vi "publishSummaryStateEvent.vi"(8 "error in (no error)":errorcluster, 11 "Model in":refnum<class "Model.lvclass">) -> (0 "error out":errorcluster, 3 "Model out":refnum<class "Model.lvclass">)   [LabVIEW 2016, in "Model.lvclass"]
uses:
  Model.lvclass
  Communicator/Topics/EventSummaryState.ctl
  Types/Timestamp.ctl
  Types/SummaryStates.ctl
  Model.lvclass/Model.ctl
  Communicator/Communicator/Communicator.lvclass
  Types/M1M3SupportTypes.lvlib
  Communicator/M1M3Communicator.lvlib
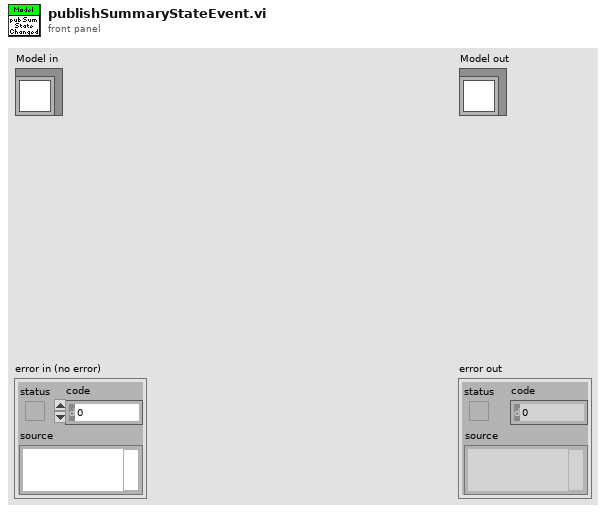
[diagram p1: front panel]
types:
  T1 = typedef "M1M3Communicator.lvlib/EventSummaryState.ctl" = cluster{"Timestamp":T2, "SummaryStates":T3}
  T2 = typedef "M1M3SupportTypes.lvlib/Timestamp.ctl" = dbl
  T3 = typedef "M1M3SupportTypes.lvlib/SummaryStates.ctl" = enum16{"OfflineState", "StandbyState", "DisabledState", "EnabledState", "FaultState"}
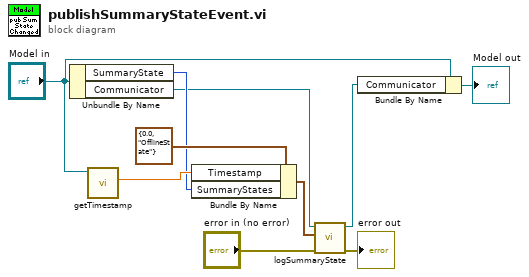
[diagram p0: block diagram]
diagram:
  n1 = Unbundle By Name("Model in") -> ("SummaryState"=w8:T3, "Communicator"=w7:refnum<class "Communicator.lvclass">)
  n2 = call "getTimestamp.vi"("Model in"="Model in") -> ("Timestamp"=w9:T2)  [unwired: 8 in, 2 out]
  n3 = Bundle By Name(cluster=T1 {"Timestamp"=0.0, "SummaryStates"=enum."OfflineState"} ("EventSummaryState"), "Timestamp"=w9, "SummaryStates"=w8) -> (w1:T1)
  n4 = call-dynamic "logSummaryState.vi"("error in (no error)"="error in (no error)", "EventSummaryState"=w1, "Communicator in"=w7) -> ("error out"=→"error out":errorcluster, "Communicator out"=w4:refnum<class "Communicator.lvclass">)  [unwired: 7 in]
  n5 = Bundle By Name(cluster="Model in", "Communicator"=w4) -> (→"Model out":refnum<class "Model.lvclass">)
